vi "Sub VI.vi"(1 "X1":dbl, 2 "X2":dbl, 3 "Y1":dbl, 4 "Y2":dbl) -> (0 "Slope":dbl)   [LabVIEW 2020]
panel:
  in  "x":dbl
  # "1)"
  # "1)"
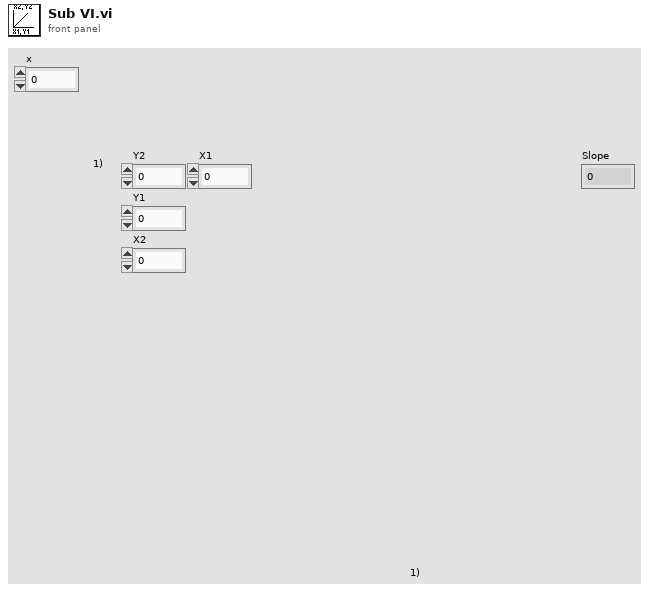
[diagram p1: front panel]
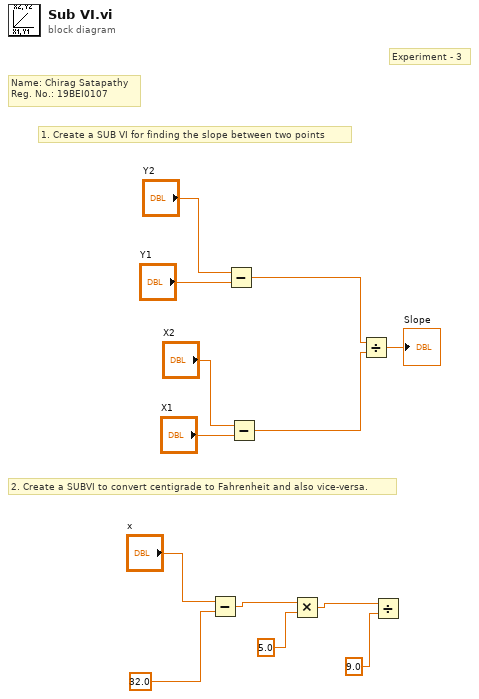
[diagram p0: block diagram]
diagram:
  # "2. Create a SUBVI to convert centigrade to Fahrenheit and also vice-versa."
  # "Name: Chirag Satapathy\nReg. No.: 19BEI0107"
  # "Experiment - 3"
  # "1. Create a SUB VI for finding the slope between two points"
  n1 = Subtract(x="x", y=32.0) -> (x-y=w4:dbl)
  n2 = Subtract(x="Y2", y="Y1") -> (x-y=w13:dbl)
  n3 = Subtract(x="X2", y="X1") -> (x-y=w12:dbl)
  n4 = Multiply(x=w4, y=5.0) -> (x*y=w2:dbl)
  n5 = Divide(x=w13, y=w12) -> (x/y=→"Slope":dbl)
  n6 = Divide(x=w2, y=9.0) -> ()  [unwired: 1 out]
